vi "COMI Get Avail Dev List.vi"(11 "pDevList":T1) -> (2 "function return":i32, 3 "pDevList out":T1)   [LabVIEW 2017, in "Comidll.lvlib"]
doc: "int (COMI_GetAvailDevList) (TComiDevList *pDevList);"
uses:
  <userlib>/Comidll/Comidll.lvlib
  <userlib>/Comidll/Comidll.dll
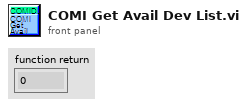
[diagram p1: front panel]
types:
  T1 = cluster{"nNumDev":u16, "@dummy control@":i8, "@dummy control@":i8, "TComiDevInfo[0]":cluster{"wSubSysID":u16, "nInstance":u32, "szDevName[0]":i8, "szDevName[1]":i8, "szDevName[2]":i8, "szDevName[3]":i8, "szDevName[4]":i8, "szDevName[5]":i8, "szDevName[6]":i8, "szDevName[7]":i8, "szDevName[8]":i8, "szDevName[9]":i8, "szDevName[10]":i8, "szDevName[11]":i8, "szDevName[12]":i8, "szDevName[13]":i8, "szDevName[14]":i8, "szDevName[15]":i8, "szDevName[16]":i8, "szDevName[17]":i8, "szDevName[18]":i8, "szDevName[19]":i8, "bDevCaps":u8, "nNumAdChan":u8}, "TComiDevInfo[1]":cluster{"wSubSysID":u16, "nInstance":u32, "szDevName[0]":i8, "szDevName[1]":i8, "szDevName[2]":i8, "szDevName[3]":i8, "szDevName[4]":i8, "szDevName[5]":i8, "szDevName[6]":i8, "szDevName[7]":i8, "szDevName[8]":i8, "szDevName[9]":i8, "szDevName[10]":i8, "szDevName[11]":i8, "szDevName[12]":i8, "szDevName[13]":i8, "szDevName[14]":i8, "szDevName[15]":i8, "szDevName[16]":i8, "szDevName[17]":i8, "szDevName[18]":i8, "szDevName[19]":i8, "bDevCaps":u8, "nNumAdChan":u8}, "TComiDevInfo[2]":cluster{"wSubSysID":u16, "nInstance":u32, "szDevName[0]":i8, "szDevName[1]":i8, "szDevName[2]":i8, "szDevName[3]":i8, "szDevName[4]":i8, "szDevName[5]":i8, "szDevName[6]":i8, "szDevName[7]":i8, "szDevName[8]":i8, "szDevName[9]":i8, "szDevName[10]":i8, "szDevName[11]":i8, "szDevName[12]":i8, "szDevName[13]":i8, "szDevName[14]":i8, "szDevName[15]":i8, "szDevName[16]":i8, "szDevName[17]":i8, "szDevName[18]":i8, "szDevName[19]":i8, "bDevCaps":u8, "nNumAdChan":u8}, "TComiDevInfo[3]":cluster{"wSubSysID":u16, "nInstance":u32, "szDevName[0]":i8, "szDevName[1]":i8, "szDevName[2]":i8, "szDevName[3]":i8, "szDevName[4]":i8, "szDevName[5]":i8, "szDevName[6]":i8, "szDevName[7]":i8, "szDevName[8]":i8, "szDevName[9]":i8, "szDevName[10]":i8, "szDevName[11]":i8, "szDevName[12]":i8, "szDevName[13]":i8, "szDevName[14]":i8, "szDevName[15]":i8, "szDevName[16]":i8, "szDevName[17]":i8, "szDevName[18]":i8, "szDevName[19]":i8, "bDevCaps":u8, "nNumAdChan":u8}, "TComiDevInfo[4]":cluster{"wSubSysID":u16, "nInstance":u32, "szDevName[0]":i8, "szDevName[1]":i8, "szDevName[2]":i8, "szDevName[3]":i8, "szDevName[4]":i8, "szDevName[5]":i8, "szDevName[6]":i8, "szDevName[7]":i8, "szDevName[8]":i8, "szDevName[9]":i8, "szDevName[10]":i8, "szDevName[11]":i8, "szDevName[12]":i8, "szDevName[13]":i8, "szDevName[14]":i8, "szDevName[15]":i8, "szDevName[16]":i8, "szDevName[17]":i8, "szDevName[18]":i8, "szDevName[19]":i8, "bDevCaps":u8, "nNumAdChan":u8}, "TComiDevInfo[5]":cluster{"wSubSysID":u16, "nInstance":u32, "szDevName[0]":i8, "szDevName[1]":i8, "szDevName[2]":i8, "szDevName[3]":i8, "szDevName[4]":i8, "szDevName[5]":i8, "szDevName[6]":i8, "szDevName[7]":i8, "szDevName[8]":i8, "szDevName[9]":i8, "szDevName[10]":i8, "szDevName[11]":i8, "szDevName[12]":i8, "szDevName[13]":i8, "szDevName[14]":i8, "szDevName[15]":i8, "szDevName[16]":i8, "szDevName[17]":i8, "szDevName[18]":i8, "szDevName[19]":i8, "bDevCaps":u8, "nNumAdChan":u8}, "TComiDevInfo[6]":cluster{"wSubSysID":u16, "nInstance":u32, "szDevName[0]":i8, "szDevName[1]":i8, "szDevName[2]":i8, "szDevName[3]":i8, "szDevName[4]":i8, "szDevName[5]":i8, "szDevName[6]":i8, "szDevName[7]":i8, "szDevName[8]":i8, "szDevName[9]":i8, "szDevName[10]":i8, "szDevName[11]":i8, "szDevName[12]":i8, "szDevName[13]":i8, "szDevName[14]":i8, "szDevName[15]":i8, "szDevName[16]":i8, "szDevName[17]":i8, "szDevName[18]":i8, "szDevName[19]":i8, "bDevCaps":u8, "nNumAdChan":u8}, "TComiDevInfo[7]":cluster{"wSubSysID":u16, "nInstance":u32, "szDevName[0]":i8, "szDevName[1]":i8, "szDevName[2]":i8, "szDevName[3]":i8, "szDevName[4]":i8, "szDevName[5]":i8, "szDevName[6]":i8, "szDevName[7]":i8, "szDevName[8]":i8, "szDevName[9]":i8, "szDevName[10]":i8, "szDevName[11]":i8, "szDevName[12]":i8, "szDevName[13]":i8, "szDevName[14]":i8, "szDevName[15]":i8, "szDevName[16]":i8, "szDevName[17]":i8, "szDevName[18]":i8, "szDevName[19]":i8, "bDevCaps":u8, "nNumAdChan":u8}, "TComiDevInfo[8]":cluster{"wSubSysID":u16, "nInstance":u32, "szDevName[0]":i8, "szDevName[1]":i8, "szDevName[2]":i8, "szDevName[3]":i8, "szDevName[4]":i8, "szDevName[5]":i8, "szDevName[6]":i8, "szDevName[7]":i8, "szDevName[8]":i8, "szDevName[9]":i8, "szDevName[10]":i8, "szDevName[11]":i8, "szDevName[12]":i8, "szDevName[13]":i8, "szDevName[14]":i8, "szDevName[15]":i8, "szDevName[16]":i8, "szDevName[17]":i8, "szDevName[18]":i8, "szDevName[19]":i8, "bDevCaps":u8, "nNumAdChan":u8}, "TComiDevInfo[9]":cluster{"wSubSysID":u16, "nInstance":u32, "szDevName[0]":i8, "szDevName[1]":i8, "szDevName[2]":i8, "szDevName[3]":i8, "szDevName[4]":i8, "szDevName[5]":i8, "szDevName[6]":i8, "szDevName[7]":i8, "szDevName[8]":i8, "szDevName[9]":i8, "szDevName[10]":i8, "szDevName[11]":i8, "szDevName[12]":i8, "szDevName[13]":i8, "szDevName[14]":i8, "szDevName[15]":i8, "szDevName[16]":i8, "szDevName[17]":i8, "szDevName[18]":i8, "szDevName[19]":i8, "bDevCaps":u8, "nNumAdChan":u8}, "TComiDevInfo[10]":cluster{"wSubSysID":u16, "nInstance":u32, "szDevName[0]":i8, "szDevName[1]":i8, "szDevName[2]":i8, "szDevName[3]":i8, "szDevName[4]":i8, "szDevName[5]":i8, "szDevName[6]":i8, "szDevName[7]":i8, "szDevName[8]":i8, "szDevName[9]":i8, "szDevName[10]":i8, "szDevName[11]":i8, "szDevName[12]":i8, "szDevName[13]":i8, "szDevName[14]":i8, "szDevName[15]":i8, "szDevName[16]":i8, "szDevName[17]":i8, "szDevName[18]":i8, "szDevName[19]":i8, "bDevCaps":u8, "nNumAdChan":u8}, "TComiDevInfo[11]":cluster{"wSubSysID":u16, "nInstance":u32, "szDevName[0]":i8, "szDevName[1]":i8, "szDevName[2]":i8, "szDevName[3]":i8, "szDevName[4]":i8, "szDevName[5]":i8, "szDevName[6]":i8, "szDevName[7]":i8, "szDevName[8]":i8, "szDevName[9]":i8, "szDevName[10]":i8, "szDevName[11]":i8, "szDevName[12]":i8, "szDevName[13]":i8, "szDevName[14]":i8, "szDevName[15]":i8, "szDevName[16]":i8, "szDevName[17]":i8, "szDevName[18]":i8, "szDevName[19]":i8, "bDevCaps":u8, "nNumAdChan":u8}, "TComiDevInfo[12]":cluster{"wSubSysID":u16, "nInstance":u32, "szDevName[0]":i8, "szDevName[1]":i8, "szDevName[2]":i8, "szDevName[3]":i8, "szDevName[4]":i8, "szDevName[5]":i8, "szDevName[6]":i8, "szDevName[7]":i8, "szDevName[8]":i8, "szDevName[9]":i8, "szDevName[10]":i8, "szDevName[11]":i8, "szDevName[12]":i8, "szDevName[13]":i8, "szDevName[14]":i8, "szDevName[15]":i8, "szDevName[16]":i8, "szDevName[17]":i8, "szDevName[18]":i8, "szDevName[19]":i8, "bDevCaps":u8, "nNumAdChan":u8}, "TComiDevInfo[13]":cluster{"wSubSysID":u16, "nInstance":u32, "szDevName[0]":i8, "szDevName[1]":i8, "szDevName[2]":i8, "szDevName[3]":i8, "szDevName[4]":i8, "szDevName[5]":i8, "szDevName[6]":i8, "szDevName[7]":i8, "szDevName[8]":i8, "szDevName[9]":i8, "szDevName[10]":i8, "szDevName[11]":i8, "szDevName[12]":i8, "szDevName[13]":i8, "szDevName[14]":i8, "szDevName[15]":i8, "szDevName[16]":i8, "szDevName[17]":i8, "szDevName[18]":i8, "szDevName[19]":i8, "bDevCaps":u8, "nNumAdChan":u8}, "TComiDevInfo[14]":cluster{"wSubSysID":u16, "nInstance":u32, "szDevName[0]":i8, "szDevName[1]":i8, "szDevName[2]":i8, "szDevName[3]":i8, "szDevName[4]":i8, "szDevName[5]":i8, "szDevName[6]":i8, "szDevName[7]":i8, "szDevName[8]":i8, "szDevName[9]":i8, "szDevName[10]":i8, "szDevName[11]":i8, "szDevName[12]":i8, "szDevName[13]":i8, "szDevName[14]":i8, "szDevName[15]":i8, "szDevName[16]":i8, "szDevName[17]":i8, "szDevName[18]":i8, "szDevName[19]":i8, "bDevCaps":u8, "nNumAdChan":u8}, "TComiDevInfo[15]":cluster{"wSubSysID":u16, "nInstance":u32, "szDevName[0]":i8, "szDevName[1]":i8, "szDevName[2]":i8, "szDevName[3]":i8, "szDevName[4]":i8, "szDevName[5]":i8, "szDevName[6]":i8, "szDevName[7]":i8, "szDevName[8]":i8, "szDevName[9]":i8, "szDevName[10]":i8, "szDevName[11]":i8, "szDevName[12]":i8, "szDevName[13]":i8, "szDevName[14]":i8, "szDevName[15]":i8, "szDevName[16]":i8, "szDevName[17]":i8, "szDevName[18]":i8, "szDevName[19]":i8, "bDevCaps":u8, "nNumAdChan":u8}}
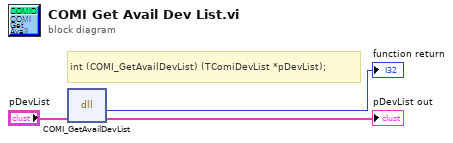
[diagram p0: block diagram]
diagram:
  # "int\t(COMI_GetAvailDevList) (TComiDevList *pDevList);"
  n1 = dll-call lib="C:/Program Files/National Instruments/LabVIEW 2017/user.lib/Comidll/Comidll.*" fn="COMI_GetAvailDevList"("pDevList"="pDevList") -> (→"function return":i32, "pDevList"=→"pDevList out":T1)  [unwired: 3 in, 2 out]
